vi "Tool ID holder.vi"(1 "Action(GET)":enum16{"GET", "SET"}(ring), 7 "value in":T1 {"LEIN implementation code" format="%.0x"; "Serial number" format="%04.0f"; "HW REV" format="%02x"}, 11 "error in (no error)":errorcluster) -> (8 "value out":T1 {"LEIN implementation code" format="%.0x"; "Serial number" format="%04.0f"; "HW REV" format="%02x"}, 15 "error out":errorcluster)   [LabVIEW 2011]
uses:
  LEINmaster/Defenitions/LEIN STAT 15 Id system cluster v2 wo lables.ctl
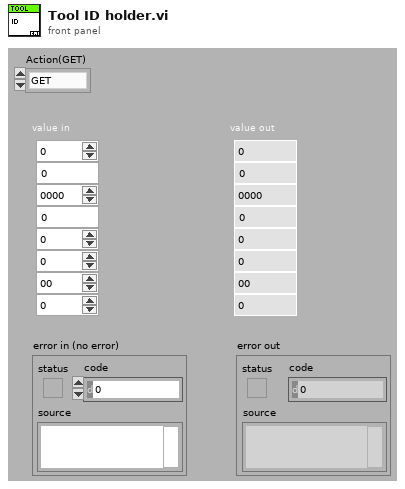
[diagram p1: front panel]
types:
  T1 = typedef "LEIN STAT 15 Id system cluster v2 wo lables.ctl" = cluster{"LEIN version":u8, "LEIN implementation code":u8, "Serial number":u16, "Project":u16, "HW ID":u8, "FW ID":u8, "HW REV":u8, "FW REV":u8}
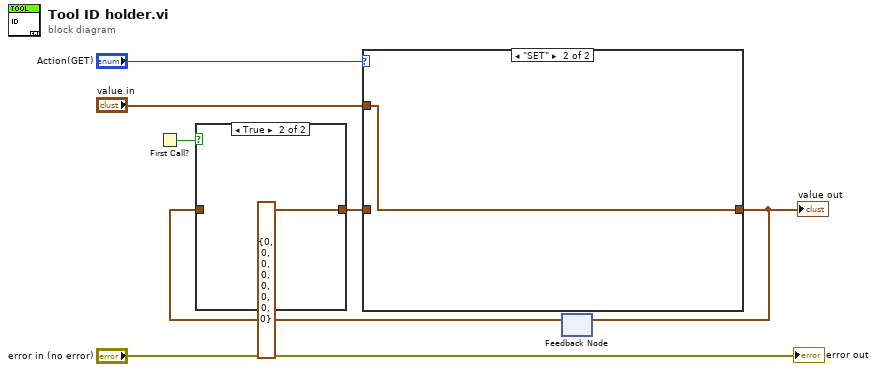
[diagram p0: block diagram]
diagram:
  n1 = First Call?() -> (First Call?: T/F=w4:bool)
  n2 = feedback #1() -> (w5:T1)  [unwired: 1 in]
  n3 = case shown="True" w4 {
    tunnel: w5 -> [w8 _]
    tunnel: [w8 T1 {"LEIN version"=0, "LEIN implementation code"=0, "Serial number"=0, "Project"=0, "HW ID"=0, "FW ID"=0, "HW REV"=0, "FW REV"=0} ("value")] -> w2
    frame False {
    }
    frame True {
    }
  }
  n4 = case shown="\"SET\"" "Action(GET)" {
    tunnel: [w10 w11] -> w3
    tunnel: w2 -> [w10 _]
    tunnel: "value in" -> [_ w11]
    frame "GET", Default {
    }
    frame "SET" {
    }
  }
  "value out" <- w3
  n5 = feedback-in #1(w3) -> ()
  "error out" <- "error in (no error)"
